vi "Test CML UI API.vi"() -> ()   [LabVIEW 2016]
doc: "CML UI API Tester.\n_____\nBased on DQMH Project Template 6.1.0.94."
uses:
  <vilib>/Utility/error.llb/DialogType.ctl
  CML UI.lvlib
panel:
  in  "Show Diagram on Init":bool
  out "error out":errorcluster
  in  "Show Block Diagram":bool
  in  "Stop Module":bool
  in  "Start Module":bool
  in  "Hide Module Panel":bool
  in  "Show Module Panel":bool
  out "Status":string
  out "Module Running?":bool
  # "This VI tests the API for the Module."
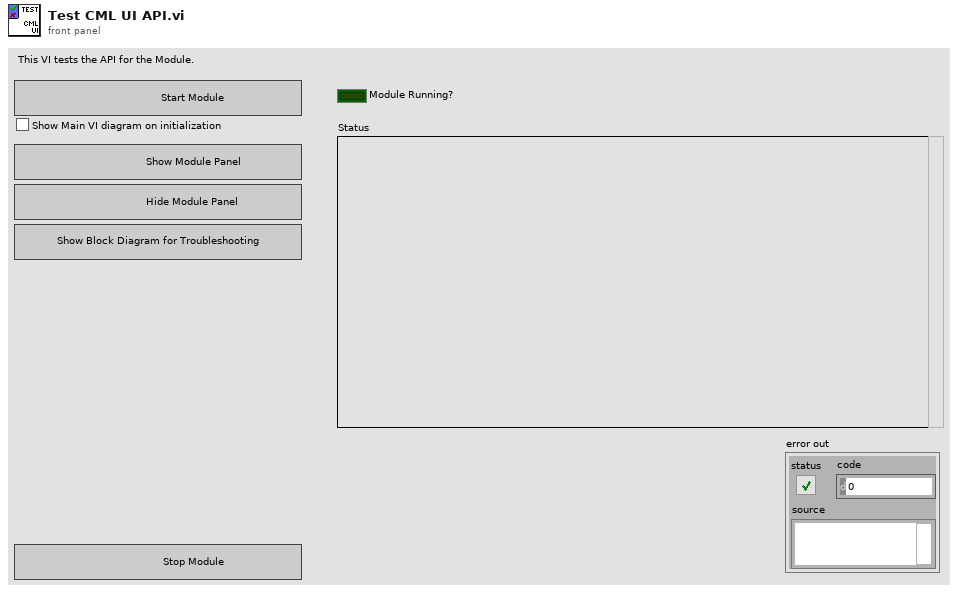
[diagram p1: front panel]
types:
  T1 = typedef "CML UI.lvlib/Broadcast Events--cluster.ctl" = cluster{"Module Did Init":refnum<user-event>, "Status Updated":refnum<user-event>, "Error Reported":refnum<user-event>, "Module Did Stop":refnum<user-event>, "Update Module Execution Status":refnum<user-event>}
  T2 = typedef "DialogType.ctl" = u16
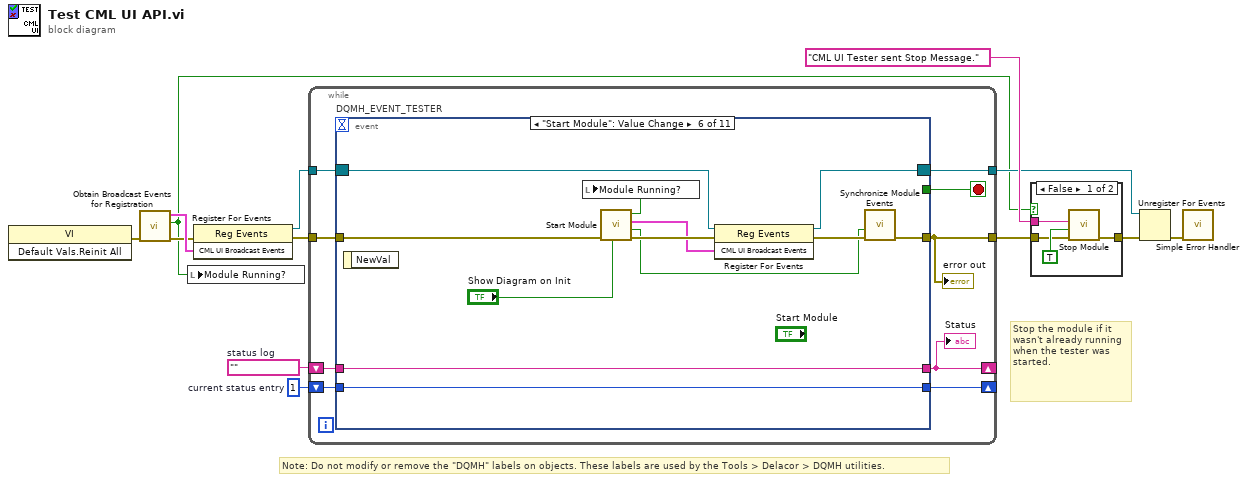
[diagram p0: block diagram]
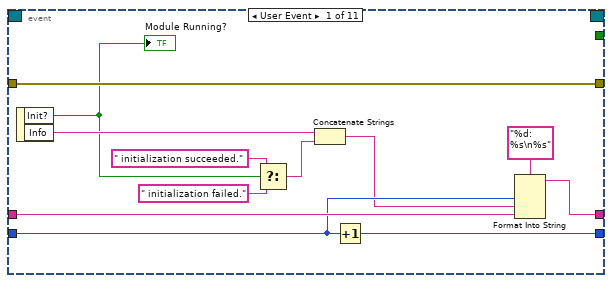
[diagram p2: hidden frame]
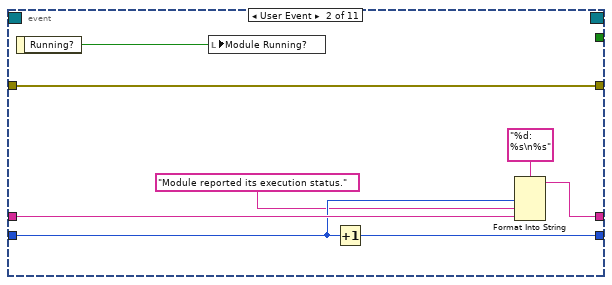
[diagram p3: hidden frame]
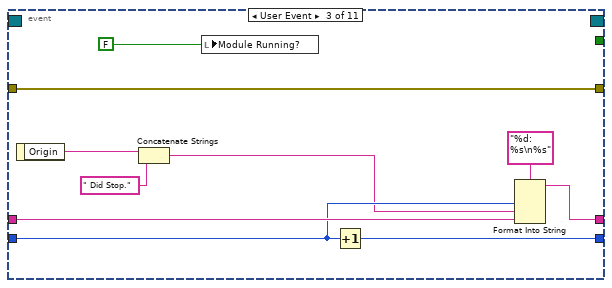
[diagram p4: hidden frame]
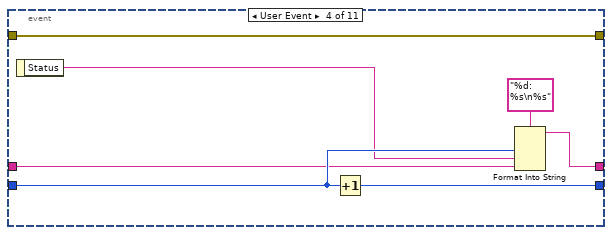
[diagram p5: hidden frame]
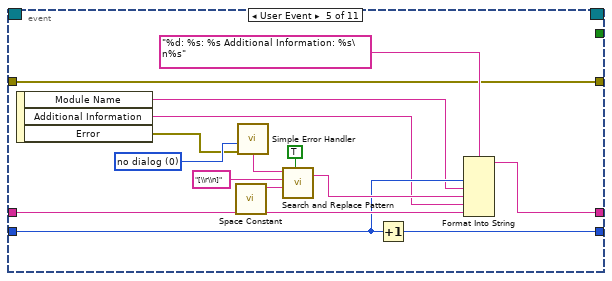
[diagram p6: hidden frame]
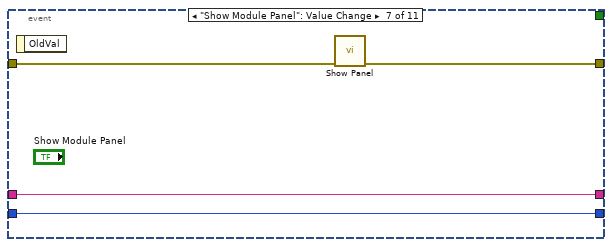
[diagram p7: hidden frame]
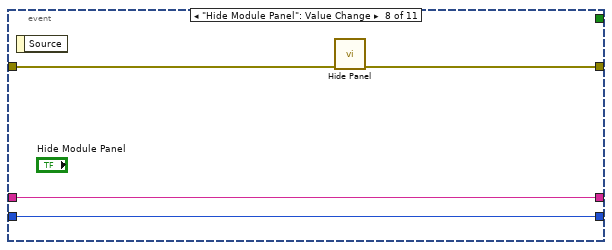
[diagram p8: hidden frame]
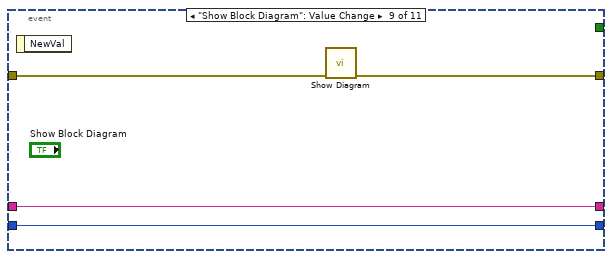
[diagram p9: hidden frame]
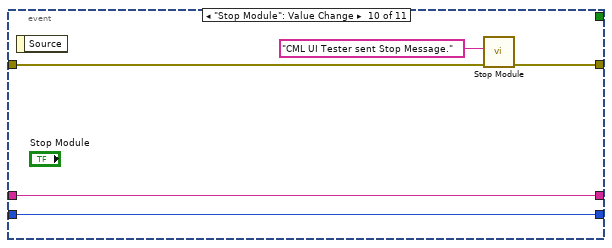
[diagram p10: hidden frame]
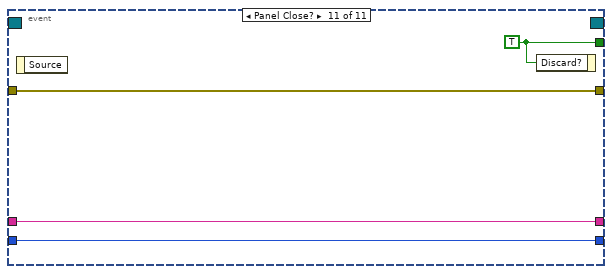
[diagram p11: hidden frame]
diagram:
  w10 = 1  # current status entry
  w11 = ""  # status log
  # "Stop the module if it wasn't already running when the tester was started."
  # "Note: Do not modify or remove the \"DQMH\" labels on objects. These labels are used by the Tools > Delacor > DQMH utilities."
  n1 = invoke class="VI" method="Default Vals.Reinit All"() -> (error out=w5:errorcluster)  [unwired: 3 in, 2 out]
  n2 = call "Obtain Broadcast Events for Registration.vi"("error in"=w5) -> ("error out"=w4:errorcluster, "Already running?"=w3:bool, "CML UI Broadcast Events"=w8:T1)  [unwired: 8 in]
  n3 = local write "Module Running?"(w3) -> ()
  n4 = register-events(error in=w4, w8) -> (reference out=w7:refnum<event-registration>, error out=w9:errorcluster)  [unwired: 1 in]
  n5 = while {
    tunnel: w7 -> [w22]
    tunnel: [w15] -> w2
    shift-right: [w18] -> _
    shift-left: w11 -> [w20]
    shift-right: [w19] -> _
    shift-left: w10 -> [w21]
    tunnel: w9 -> [w17]
    tunnel: [w16] -> w6
    stop <- w14 stop-if-true
    n6 = event "DQMH_EVENT_TESTER" shown="[5] \"Start Module\": Value Change" {
      selector: w22 -> [_ _ _ _ _ w80 _ _ _ _ _]
      dyn-events: [_ _ _ _ _ w79 _ _ _ _ _] -> w16
      timeout: _ -> [_ _ _ _ _ _ _ _ _ _ _]
      tunnel: [_ _ _ _ _ _ _ _ _ _ w107] -> w14
      tunnel: [w34 w36 w43 w53 w63 w78 w90 w94 w95 w101 w104] -> w15
      tunnel: w21 -> [w31 w40 w50 w56 w66 w83 w88 w92 w96 w102 w105]
      tunnel: w20 -> [w32 w41 w51 w55 w67 w84 w89 w93 w97 w103 w106]
      tunnel: [w29 w38 w48 w57 w65 w84 w89 w93 w97 w103 w106] -> w18
      tunnel: [w30 w39 w49 w59 w64 w83 w88 w92 w96 w102 w105] -> w19
      tunnel: w17 -> [w34 w36 w43 w53 w63 w77 w87 w91 w98 w99 w104]
      event User Event {
        n7 = event-data() -> ("Init?"=w26:bool, "Info"=w28:string)  [unwired: 1 in]
        "Module Running?" <- w26
        n8 = Select(t=" initialization succeeded.", s=w26, f=" initialization failed.") -> (s? t:f=w23:string)
        n9 = Concatenate Strings(w28, w23) -> (w27:string)
        n10 = Increment(x=w31) -> (x+1=w30:i32)
        n11 = Format Into String(format string="%d: %s\n%s", w31, w27, w32) -> (resulting string=w29:string)  [unwired: 2 in, 1 out]
      }
      event User Event {
        n12 = event-data() -> ("Running?"=w35:bool)  [unwired: 1 in]
        n13 = local write "Module Running?"(w35) -> ()
        n14 = Increment(x=w40) -> (x+1=w39:i32)
        n15 = Format Into String(format string="%d: %s\n%s", w40, "Module reported its execution status.", w41) -> (resulting string=w38:string)  [unwired: 2 in, 1 out]
      }
      event User Event {
        n16 = event-data() -> ("Origin"=w47:string)  [unwired: 1 in]
        n17 = Concatenate Strings(w47, " Did Stop.") -> (w46:string)
        n18 = local write "Module Running?"(FALSE ("Module Did Init?")) -> ()
        n19 = Increment(x=w50) -> (x+1=w49:i32)
        n20 = Format Into String(format string="%d: %s\n%s", w50, w46, w51) -> (resulting string=w48:string)  [unwired: 2 in, 1 out]
      }
      event User Event {
        n21 = event-data() -> ("Status"=w54:string)  [unwired: 1 in]
        n22 = Increment(x=w56) -> (x+1=w59:i32)
        n23 = Format Into String(format string="%d: %s\n%s", w56, w54, w55) -> (resulting string=w57:string)  [unwired: 2 in, 1 out]
      }
      event User Event {
        w68 = T2 0 items=["no dialog", "OK message", "continue or stop message", "OK message + warnings", "continue/stop + warnings"] ("type of dialog (OK msg:1)")
        n24 = event-data() -> ("Module Name"=w62:string, "Additional Information"=w61:string, "Error"=w60:errorcluster)  [unwired: 1 in]
        n25 = call <vilib>:"Space Constant.vi"() -> ("String"=w72:string)
        n26 = call <vilib>:"Simple Error Handler.vi"("type of dialog (OK msg:1)"=w68, "error in (no error)"=w60) -> ("message"=w69:string)  [unwired: 3 in, 4 out]
        n27 = call <vilib>:"Search and Replace Pattern.vi"("string"=w69, "regular expression (\"\")"="[\\r\\n]" ("regular expression (\"\")"), "replace string (\"\")"=w72, "replace all? (F)"=TRUE ("replace all CR/LF with spaces")) -> ("result string"=w70:string)  [unwired: 1 in, 1 out]
        n28 = Increment(x=w66) -> (x+1=w64:i32)
        n29 = Format Into String(format string="%d: %s: %s Additional Information: %s\n%s", w66, w62, w70, w61, w67) -> (resulting string=w65:string)  [unwired: 2 in, 1 out]
      }
      event "Start Module": Value Change {
        n30 = event-data() -> ()  [unwired: 1 in, 1 out]
        n31 = call "Start Module.vi"("Show Main VI Diagram on Init (F)"="Show Diagram on Init", "error in"=w77) -> ("error out"=w85:errorcluster, "Wait for Event Sync?"=w82:bool, "CML UI Broadcast Events"=w81:T1, "Module Was Already Running?"=w76:bool)  [unwired: 6 in]
        n32 = local write "Module Running?"(w76) -> ()
        n33 = register-events(reference=w80, error in=w85, w81) -> (reference out=w79:refnum<event-registration>, error out=w86:errorcluster)
        n34 = call "Synchronize Module Events.vi"("error in (no error)"=w86, "Wait for Event Sync?"=w82) -> ("error out"=w78:errorcluster)  [unwired: 9 in]
      }
      event "Show Module Panel": Value Change {
        n35 = event-data() -> ()  [unwired: 1 in, 1 out]
        n36 = call "Show Panel.vi"("error in (no error)"=w87) -> ("error out"=w90:errorcluster)  [unwired: 10 in]
      }
      event "Hide Module Panel": Value Change {
        n37 = event-data() -> ()  [unwired: 1 in, 1 out]
        n38 = call "Hide Panel.vi"("error in (no error)"=w91) -> ("error out"=w94:errorcluster)  [unwired: 10 in]
      }
      event "Show Block Diagram": Value Change {
        n39 = event-data() -> ()  [unwired: 1 in, 1 out]
        n40 = call "Show Diagram.vi"("error in (no error)"=w98) -> ("error out"=w95:errorcluster)  [unwired: 10 in]
      }
      event "Stop Module": Value Change {
        n41 = event-data() -> ()  [unwired: 1 in, 1 out]
        n42 = call "Stop Module.vi"("error in"=w99, "Origin"="CML UI Tester sent Stop Message.") -> ("error out"=w101:errorcluster)  [unwired: 9 in]
      }
      event Panel Close? {
        w107 = TRUE ("Discard?")
        n43 = event-data() -> ()  [unwired: 1 in, 1 out]
        n44 = event-data("Discard?"=w107) -> ()  [unwired: 1 in, 1 out]
      }
    }
    "Status" <- w18
    "error out" <- w15
  }
  n45 = case shown="False" w3 {
    tunnel: [w111 w112] -> w13
    tunnel: "CML UI Tester sent Stop Message." ("Origin") -> [w110 _]
    tunnel: w2 -> [w108 w112]
    frame False {
      n46 = call "Stop Module.vi"("error in"=w108, "Wait for Module to Stop? (F)"=TRUE ("Wait for Module to stop?"), "Origin"=w110) -> ("error out"=w111:errorcluster)  [unwired: 8 in]
    }
    frame True {
    }
  }
  n47 = Unregister For Events(event registration refnum=w6, error in=w13) -> (error out=w1:errorcluster)
  n48 = call <vilib>:"Simple Error Handler.vi"("error in (no error)"=w1) -> ()  [unwired: 4 in, 5 out]
